vi "MS_Comm_to_Var_Binary.vi"(9 "Input Data":bool[](array[boolean]), 11 "Boolean":bool) -> ()   [LabVIEW 2016, in "DNP3_Master_Station_Template.lvlib"]
uses:
  DNP3_Master_Station_Template.lvlib
  <vilib>/Utility/file.llb/Read Delimited Spreadsheet (string).vi
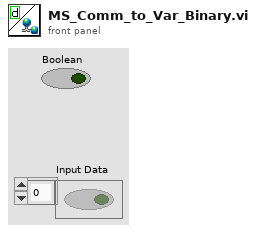
[diagram p1: front panel]
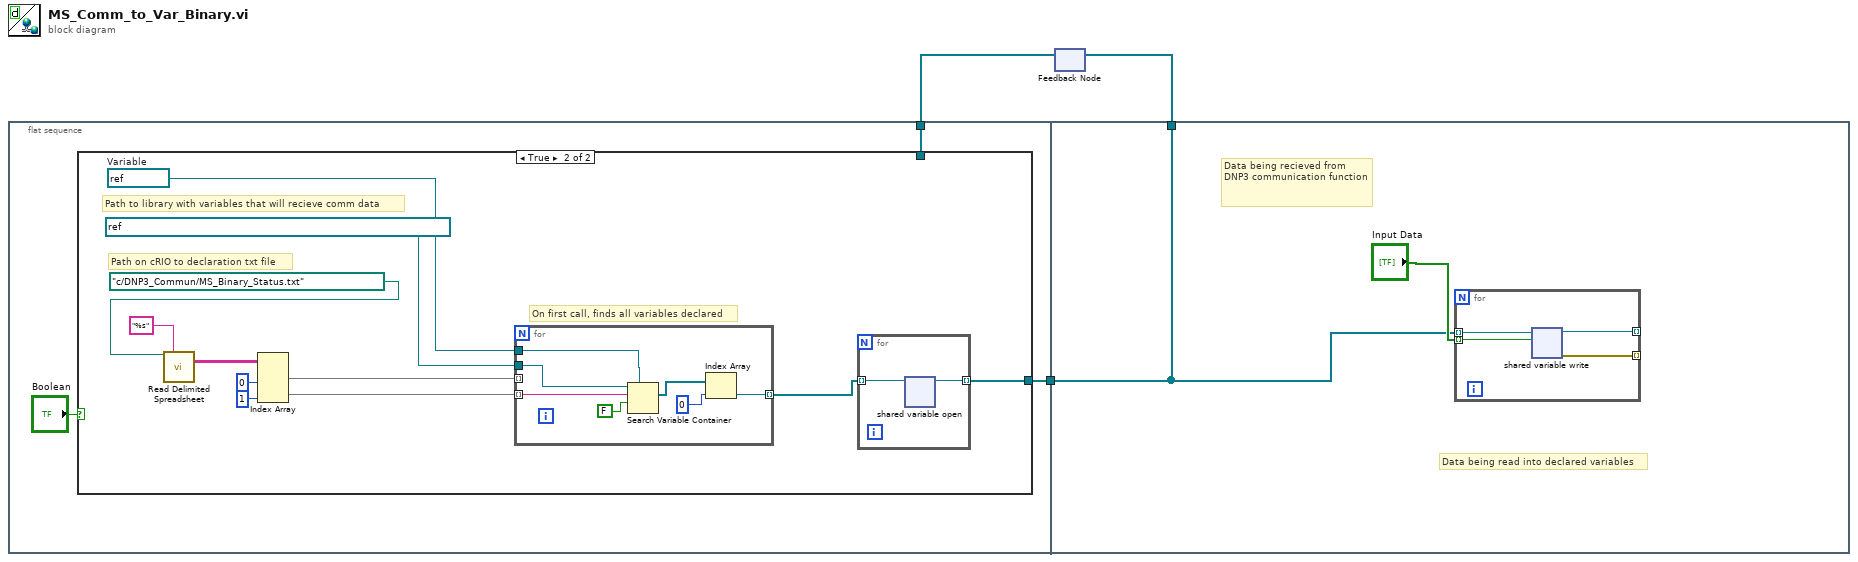
[diagram p0: block diagram]
diagram:
  n1 = flat-sequence {
    tunnel: [w6] -> w3
    tunnel: w1 -> [w5]
    tunnel: w3 -> [w28]
    tunnel: [w28] -> w2
    frame #0 {
      n2 = case shown="True" "Boolean" {
        tunnel: [w7 w9] -> w6
        tunnel: w5 -> [w7 _]
        frame False {
        }
        frame True {
          w10 = refnum<k21> refnum  # Variable
          # "On first call, finds all variables declared"
          # "Path on cRIO to declaration txt file"
          # "Path to library with variables that will recieve comm data"
          n3 = call-poly <vilib>:"Read Delimited Spreadsheet.vi"("file path (dialog if empty)"=path "c:/DNP3_Commun/MS_Binary_Status.txt" ("file path (use dialog)"), "format (%s)"="%s") -> ("all rows"=w14:string[][])  [unwired: 8 in, 5 out]
          n4 = Index Array(array=w14, index (col) #1=0 ("disabled index (col)"), index (col) #2=1 ("index (col)")) -> (element #1=w17:string[], element #2=w18:string[])  [unwired: 2 in]
          n5 = for {
            tunnel: w10 -> [w24]
            tunnel: refnum<k21> "ni.var.psp://localhost/MS_Data_Variables/MS_Binary_Status/" ("container refnum in") -> [w23]
            tunnel: w17 -> [_] mode=indexing
            tunnel: w18 -> [w22] mode=indexing
            tunnel: [w21] -> w8 mode=indexing
            n6 = Search Variable Container(7:w24, 9:FALSE, 10:w22, 11:w23) -> (2:w27:refnum<k21>[])  [unwired: 2 in, 2 out]
            n7 = Index Array(array=w27, index=0) -> (element=w21:refnum<k21>)
          }
          n8 = for {
            tunnel: [w20] -> w9 mode=indexing
            tunnel: w8 -> [w19] mode=indexing
            n9 = shared-variable-open(w19) -> (w20:refnum<k21>)  [unwired: 2 in, 1 out]
          }
        }
      }
    }
    frame #1 {
      # "Data being recieved from DNP3 communication function"
      # "Data being read into declared variables"
      n10 = for {
        tunnel: "Input Data" -> [w33] mode=indexing
        tunnel: w28 -> [w32] mode=indexing
        tunnel: [w31] -> _ mode=indexing
        tunnel: [w30] -> _ mode=indexing
        n11 = shared-variable-write(w32, w33) -> (w31:refnum<k21>, w30:errorcluster)  [unwired: 1 in]
      }
    }
  }
  n12 = feedback-in #1(w2) -> ()
  n13 = feedback #1() -> (w1:refnum<k21>[])  [unwired: 1 in]
